vi "respond to response.vi"(8 "error in (no error)":errorcluster caption="Fehler (Eingang, kein Fehler)", 10 "?":T1={"commandlist"="", "line"=0, "last response"="", "timeout"=0, "wait"=0, "erfolgreich"=FALSE, "next state"=enum."init", "Zustand"=enum."starting", "manual Test"=FALSE}, 11 "Burst Eingang":refnum<class "Burst.lvclass"> caption="DNL_LabVIEW Object in") -> (0 "error out":errorcluster caption="Fehler (Ausgang)", 1 "read again?":bool, 2 "?":T1={"commandlist"="", "line"=0, "last response"="", "timeout"=0, "wait"=0, "erfolgreich"=FALSE, "next state"=enum."init", "Zustand"=enum."starting", "manual Test"=FALSE}, 3 "Burst Ausgang":refnum<class "Burst.lvclass"> caption="DNL_LabVIEW Object out")   [LabVIEW 2013, in "Burst.lvclass"]
uses:
  Burst.lvclass
  Main/controls/TestData.ctl
  Main/controls/TestStates.ctl
  Main/controls/generalTestStates.ctl
  lib/EMV-Test.lvlib
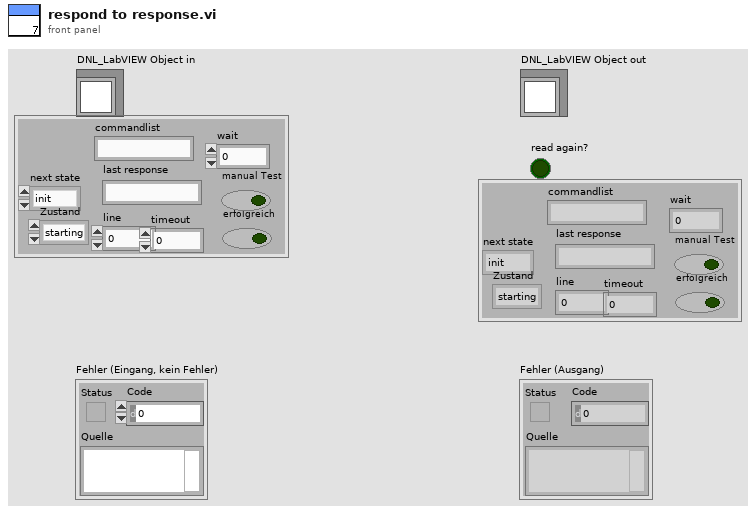
[diagram p1: front panel]
types:
  T1 = typedef "EMV-Test.lvlib/TestData.ctl" = cluster{"commandlist":string, "line":i32, "last response":string, "timeout":i32, "wait":u32, "erfolgreich":bool, "next state":T2, "Zustand":T3, "manual Test":bool}
  T2 = typedef "EMV-Test.lvlib/TestStates.ctl" = enum16{"event loop", "save Test", "Custom Action 1", "Custom Action 2", "pause", "vorgefertigter Test", "manueller Test", "respond to response", "error", "init", "start Test", "evaluate line", "wait for Response", "wait", "catch error", "close Connection", "end"}
  T3 = typedef "generalTestStates.ctl" = enum16{"paused", "starting", "waiting", "running", "finished"}
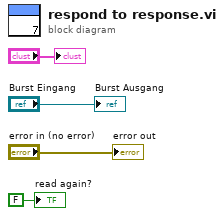
[diagram p0: block diagram]
diagram:
  "error out" <- "error in (no error)"
  "Burst Ausgang" <- "Burst Eingang"
  "read again?" <- FALSE ("read again?")
  "?" <- "?"
